vi "6-4.vi"() -> ()   [LabVIEW 2017]
uses:
  <vilib>/Utility/file.llb/Write Delimited Spreadsheet (DBL).vi
  <vilib>/measure/NI_MABase.lvlib
panel:
  out "添加的数组":dbl[][](array[numeric])
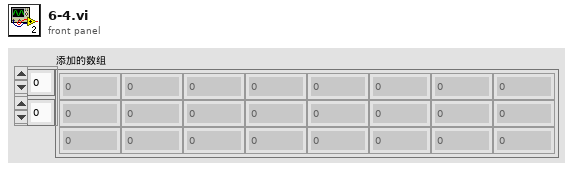
[diagram p1: front panel]
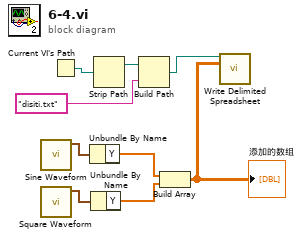
[diagram p0: block diagram]
diagram:
  n1 = call <vilib>:"Sine Waveform.vi"() -> ("signal out"=w5:waveform(dbl))  [unwired: 10 in, 1 out]
  n2 = call <vilib>:"Square Waveform.vi"() -> ("signal out"=w6:waveform(dbl))  [unwired: 10 in, 1 out]
  n3 = Current VI's Path() -> (path=w9:path)
  n4 = Unbundle By Name(w5) -> ("Y"=w4:dbl[])
  n5 = Unbundle By Name(w6) -> ("Y"=w3:dbl[])
  n6 = Strip Path(path=w9) -> (stripped path=w8:path)  [unwired: 1 out]
  n7 = Build Path(base path=w8, name or relative path="disiti.txt" ("名称或相对路径")) -> (appended path=w2:path)
  n8 = Build Array(w4, w3) -> (w1:dbl[][])
  "添加的数组" <- w1
  n9 = call-poly <vilib>:"Write Delimited Spreadsheet.vi"("file path (dialog if empty)"=w2, "2D data"=w1) -> ()  [unwired: 12 in, 2 out]
